vi "OpenConfig.vi"(8 "error in (no error)":errorcluster, 10 "create file if necessary (T)":bool=TRUE, 11 "Config File Name":string="RobotConfig.ini") -> (0 "error out":errorcluster, 2 "file created?":bool, 3 "refnum":T1)   [LabVIEW 2014]
uses:
  <vilib>/Utility/config.llb/Config Data RefNum.ctl
  <vilib>/Utility/config.llb/NI_LVConfig.lvlib
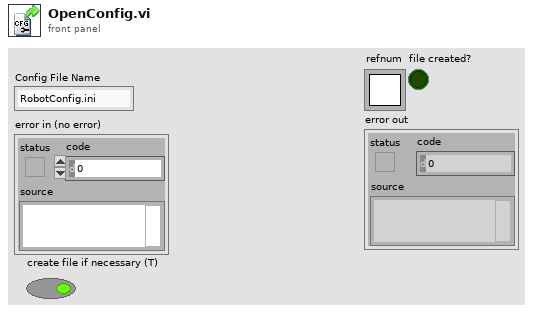
[diagram p1: front panel]
types:
  T1 = typedef "NI_LVConfig.lvlib/Config Data RefNum.ctl" = refnum<k1>
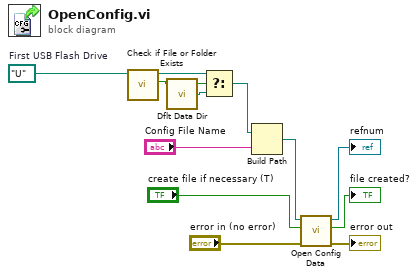
[diagram p0: block diagram]
diagram:
  w6 = path "U:/"  # First USB Flash Drive
  n1 = call <vilib>:"Check if File or Folder Exists.vi"("path"=w6) -> ("file or folder exists?"=w11:bool, "dup path"=w12:path)  [unwired: 8 in, 1 out]
  n2 = call <vilib>:"Dflt Data Dir.vi"() -> ("App:Default Data Directory"=w10:path)
  n3 = Select(t=w12, s=w11, f=w10) -> (s? t:f=w9:path)
  n4 = Build Path(base path=w9, name or relative path="Config File Name") -> (appended path=w7:path)
  n5 = call <vilib>:"Open Config Data.vi"("error in (no error)"="error in (no error)", "create file if necessary (T)"="create file if necessary (T)", "configuration file path"=w7) -> ("error out"=→"error out":errorcluster, "file created?"=→"file created?":bool, "refnum"=→"refnum":T1)  [unwired: 6 in]
